vi "update sync UI.vi"(8 "error in (no error)":errorcluster, 10 "sync ui refs":T1, 11 "shared memory editor node in":refnum<class "module editor node.lvclass">) -> (0 "error out":errorcluster, 3 "shared memory editor node out":refnum<class "module editor node.lvclass">)   [LabVIEW 2013, in "Shared Memory editor node.lvclass"]
uses:
  Shared Memory editor node.lvclass
  <vilib>/NI/DCAF/Tag Editor Core/Configuration Editor/Classes/Module editor node/module editor node.lvclass
  sync ui controls.ctl
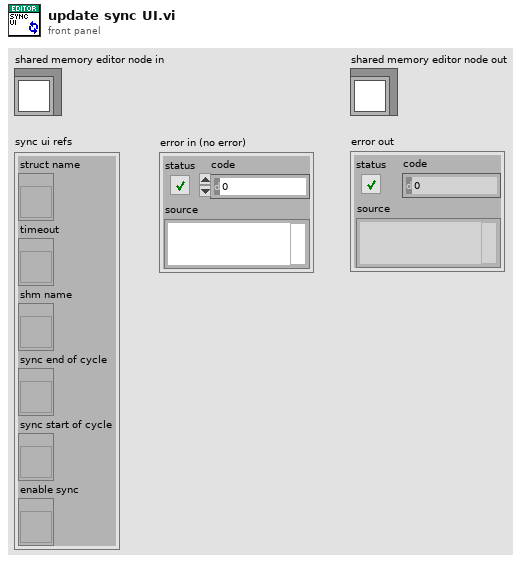
[diagram p1: front panel]
types:
  T1 = typedef "Shared Memory editor node.lvclass/sync ui controls.ctl" = cluster{"struct name":refnum<vi>, "timeout":refnum<vi>, "shm name":refnum<vi>, "sync end of cycle":refnum<vi>, "sync start of cycle":refnum<vi>, "enable sync":refnum<vi>}
  T2 = typedef "Shared Memory configuration.lvclass/sync item.ctl" = cluster{"mechanism":T3, "name":string}
  T3 = typedef "Shared Memory configuration.lvclass/sync mechanism.ctl" = enum16{"Semaphore"}
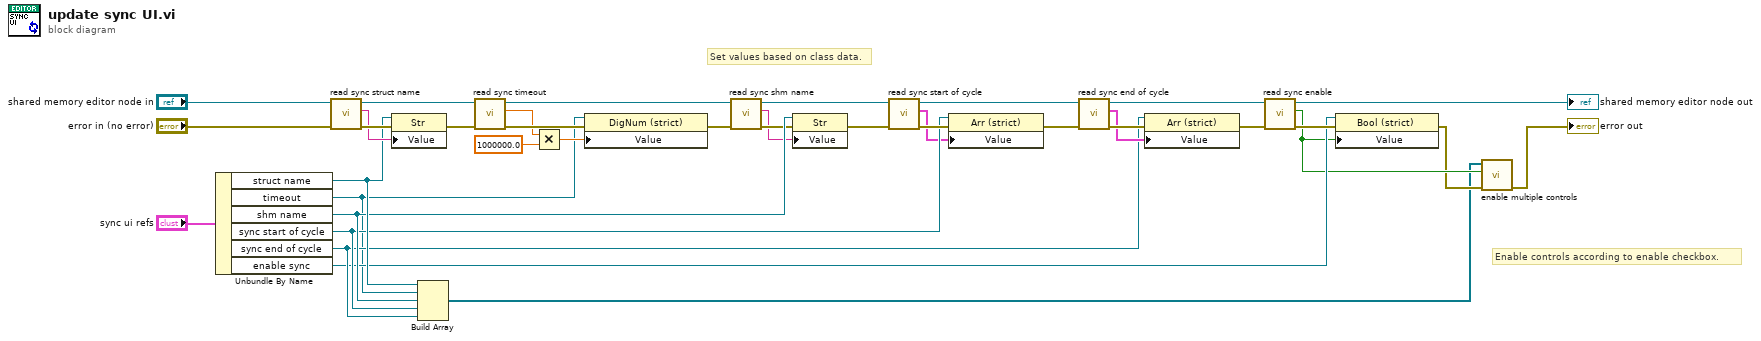
[diagram p0: block diagram]
diagram:
  # "Enable controls according to enable checkbox."
  # "Set values based on class data."
  n1 = Unbundle By Name("sync ui refs") -> ("struct name"=w24:refnum<vi>, "timeout"=w1:refnum<vi>, "shm name"=w23:refnum<vi>, "sync start of cycle"=w17:refnum<vi>, "sync end of cycle"=w9:refnum<vi>, "enable sync"=w7:refnum<vi>)
  n2 = call "read sync struct name.vi"("error in"="error in (no error)", "shared memory editor node"="shared memory editor node in") -> ("error out"=w34:errorcluster, "sync struct name"=w33:string, "shared memory editor node out"=w32:refnum<class "module editor node.lvclass">)  [unwired: 7 in]
  n3 = property class="Str"(reference=w24, error in=w34, "Value"=w33) -> (error out=w31:errorcluster)  [unwired: 1 out]
  n4 = Build Array(w24, w1, w23, w17, w9) -> (w2:refnum<vi>[])
  n5 = call "read sync timeout.vi"("error in"=w31, "shared memory editor node"=w32) -> ("error out"=w28:errorcluster, "sync struct name"=w26:dbl, "shared memory editor node out"=w27:refnum<class "module editor node.lvclass">)  [unwired: 7 in]
  n6 = Multiply(x=w26, y=1000000.0) -> (x*y=w29:dbl)
  n7 = property class="DigNum (strict)"(reference=w1, error in=w28, "Value"=w29) -> (error out=w25:errorcluster)  [unwired: 1 out]
  n8 = call "read sync shm name.vi"("error in"=w25, "shared memory editor node"=w27) -> ("error out"=w22:errorcluster, "sync shm name"=w21:string, "shared memory editor node out"=w20:refnum<class "module editor node.lvclass">)  [unwired: 7 in]
  n9 = property class="Str"(reference=w23, error in=w22, "Value"=w21) -> (error out=w19:errorcluster)  [unwired: 1 out]
  n10 = call "read sync start of cycle.vi"("error in"=w19, "shared memory editor node"=w20) -> ("error out"=w18:errorcluster, "sync start of cycle"=w16:T2[], "shared memory editor node out"=w15:refnum<class "module editor node.lvclass">)  [unwired: 7 in]
  n11 = property class="Arr (strict)"(reference=w17, error in=w18, "Value"=w16) -> (error out=w14:errorcluster)  [unwired: 1 out]
  n12 = call "read sync end of cycle.vi"("error in"=w14, "shared memory editor node"=w15) -> ("error out"=w13:errorcluster, "sync end of cycle"=w10:T2[], "shared memory editor node out"=w11:refnum<class "module editor node.lvclass">)  [unwired: 7 in]
  n13 = property class="Arr (strict)"(reference=w9, error in=w13, "Value"=w10) -> (error out=w12:errorcluster)  [unwired: 1 out]
  n14 = call "read sync enable.vi"("error in"=w12, "shared memory editor node"=w11) -> ("error out"=w8:errorcluster, "sync enable"=w6:bool, "shared memory editor node out"=→"shared memory editor node out":refnum<class "module editor node.lvclass">)  [unwired: 7 in]
  n15 = property class="Bool (strict)"(reference=w7, error in=w8, "Value"=w6) -> (error out=w5:errorcluster)  [unwired: 1 out]
  n16 = call "enable multiple controls.vi"("error in (no error)"=w5, "enabled? (T)"=w6, "controls in"=w2) -> ("error out"=→"error out":errorcluster)  [unwired: 6 in, 2 out]
